vi "p1.vi"() -> ()   [LabVIEW 2025, in "d11.lvlib"]
uses:
  d11.lvlib
  <vilib>/Utility/error.llb/Trim Whitespace One-Sided.vi
  AOC/AOC.lvlib
panel:
  in  "Example":string="aaa: you hhh\nyou: bbb ccc\nbbb: ddd eee\nccc: ddd eee fff\nddd: ggg\neee: out\nfff: out\nggg: out\nhhh: ccc fff iii\niii: out"
  in  "Example":bool
  out "Answer":i64
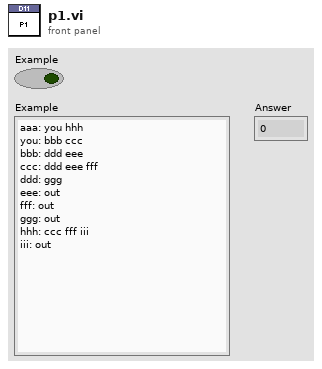
[diagram p1: front panel]
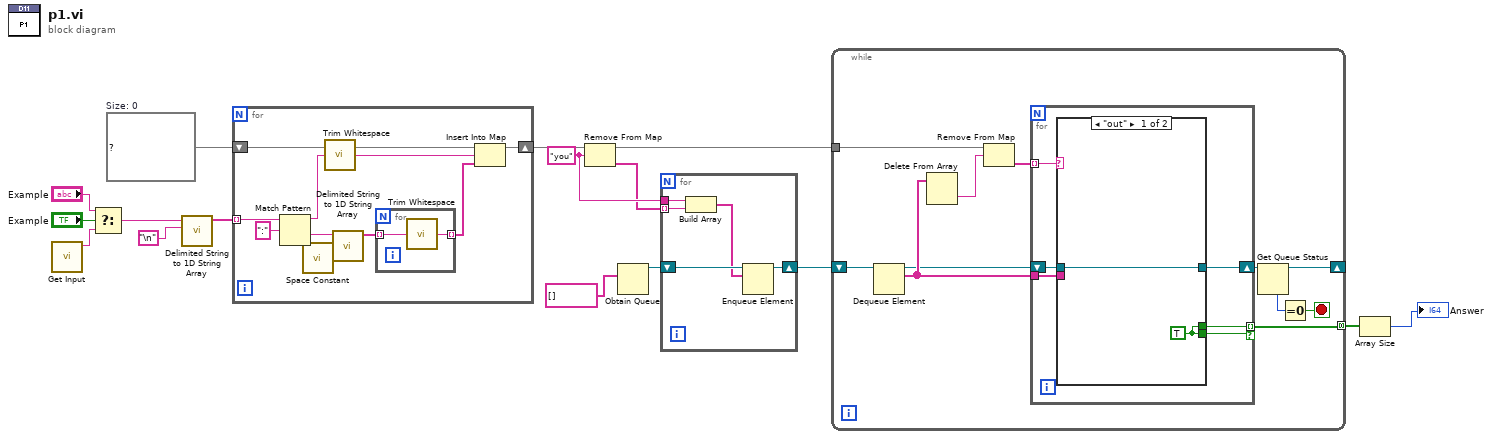
[diagram p0: block diagram]
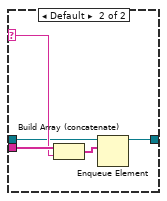
[diagram p2: hidden frame]
diagram:
  w5 = "you" ("key")
  w10 = map{string, string[]} {}  # Size: 0
  n1 = call "Get Input.vi"() -> ("Input"=w16:string)  [unwired: 11 in]
  n2 = Select(t="Example", s="Example", f=w16) -> (s? t:f=w13:string)
  n3 = call <vilib>:"Delimited String to 1D String Array.vi"("delimiter"="\n", "delimited string"=w13) -> ("string array"=w11:string[])  [unwired: 9 in]
  n4 = for {
    tunnel: w11 -> [w25] mode=indexing
    shift-right: [w17] -> w9
    shift-left: w10 -> [w26]
    n5 = Match Pattern(string=w25, regular expression=":" ("search string/char (-)")) -> (before substring=w23:string, after substring=w21:string)  [unwired: 1 in, 2 out]
    n6 = call <vilib>:"Space Constant.vi"() -> ("String"=w20:string)
    n7 = call <vilib>:"Trim Whitespace.vi"("string"=w23) -> ("trimmed string"=w22:string)  [unwired: 1 in]
    n8 = call <vilib>:"Delimited String to 1D String Array.vi"("delimiter"=w20, "delimited string"=w21) -> ("string array"=w19:string[])  [unwired: 9 in]
    n9 = for {
      tunnel: w19 -> [w28] mode=indexing
      tunnel: [w27] -> w18 mode=indexing
      n10 = call <vilib>:"Trim Whitespace.vi"("string"=w28) -> ("trimmed string"=w27:string)  [unwired: 1 in]
    }
    n11 = Insert Into Map(map in=w26, key=w22, value=w18) -> (map out=w17:map{string, string[]})  [unwired: 2 out]
  }
  n12 = Remove From Map(10:w5, 11:w9) -> (1:w4:string[], 3:w8:map{string, string[]})  [unwired: 1 out]
  n13 = Obtain Queue(element data type=string[] []) -> (queue out=w6:refnum<queue>)  [unwired: 4 in, 2 out]
  n14 = for {
    tunnel: w5 -> [w32]
    tunnel: w4 -> [w30] mode=indexing
    shift-right: [w29] -> w3
    shift-left: w6 -> [w33]
    n15 = Build Array(w32, w30) -> (w31:string[])
    n16 = Enqueue Element(queue=w33, element=w31) -> (queue out=w29:refnum<queue>)  [unwired: 2 in, 2 out]
  }
  n17 = while {
    tunnel: w8 -> [w43]
    shift-right: [w37] -> _
    shift-left: w3 -> [w44]
    tunnel: [w34] -> w1 mode=concatenating
    stop <- w35 stop-if-true
    n18 = Dequeue Element(queue=w44) -> (queue out=w39:refnum<queue>, element=w40:string[])  [unwired: 2 in, 2 out]
    n19 = Delete From Array(array=w40) -> (deleted portion=w42:string)  [unwired: 2 in, 1 out]
    n20 = Remove From Map(10:w42, 11:w43) -> (1:w41:string[])  [unwired: 2 out]
    n21 = for {
      tunnel: w41 -> [w49] mode=indexing
      tunnel: w40 -> [w50]
      shift-right: [w47] -> w38
      shift-left: w39 -> [w48]
      tunnel: [w46] -> w34 mode=indexing if=w45
      n22 = case shown="\"out\"" w49 {
        selector: w49 -> [_ w56]
        tunnel: w50 -> [_ w57]
        tunnel: w48 -> [w52 w55]
        tunnel: [w52 w53] -> w47
        tunnel: [w51 _] -> w46
        tunnel: [w51 _] -> w45
        frame "out" {
          w51 = TRUE
        }
        frame Default {
          n23 = Build Array (concatenate)(w57, w56) -> (w54:string[])
          n24 = Enqueue Element(queue=w55, element=w54) -> (queue out=w53:refnum<queue>)  [unwired: 2 in, 2 out]
        }
      }
    }
    n25 = Get Queue Status(queue=w38) -> (queue out=w37:refnum<queue>, # elements in queue=w36:i32)  [unwired: 2 in, 6 out]
    n26 = Equal To 0?(x=w36) -> (x = 0?=w35:bool)
  }
  n27 = Array Size(array=w1) -> (size(s)=→"Answer":i32)
